vi "Add Topic.vi"(8 "error in (no error)":errorcluster, 9 "Topic Enqueuer":refnum<class "Message Enqueuer.lvclass">, 10 "Topic Object":refnum<class "Topic.lvclass">, 11 "TopicLookupTable":refnum<data-value>) -> (0 "error out":errorcluster, 2 "Topic Replaced?":bool, 3 "TopicLookupTable":refnum<data-value>)   [LabVIEW 2017, in "Mediator.lvlib" / "TopicLookupTable.lvclass"]
doc: "<License>\nCopyright © 2017 Composed Systems, LLC | All rights reserved\nwww.composed.io\n\nAuthor: Ethan Stern <ethan.stern@composed.io>\n\nThis software is provided \"AS IS\" WITHOUT WARRANTIES, either express or implied, AND IS FOR EDUCATIONAL PURPOSES ONLY.\n</License>"
uses:
  TopicLookupTable.lvclass
  Topic/Topic.lvclass
  <vilib>/ActorFramework/Message Enqueuer/Message Enqueuer.lvclass
  Topic/Topic.lvclass/Topic.ctl
  TopicLookupTable.lvclass/TopicLookupTable.ctl
  <vilib>/ActorFramework/Actor/Read Self Enqueuer.vi
  <vilib>/ActorFramework/Message Enqueuer/Init from Existing Queue.vi
  <vilib>/ErrorRing/Error Ring.xnode
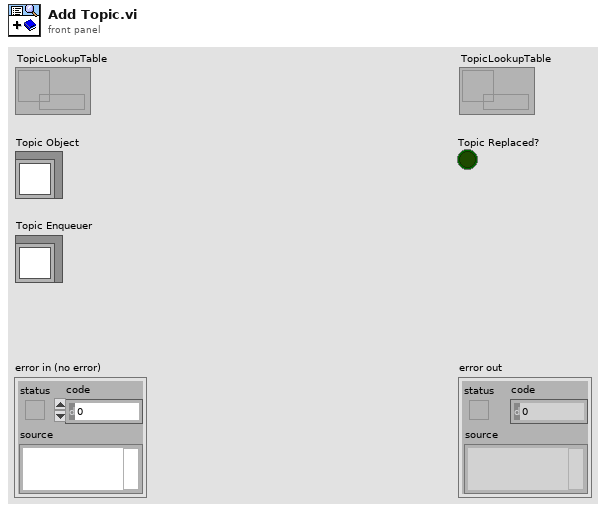
[diagram p1: front panel]
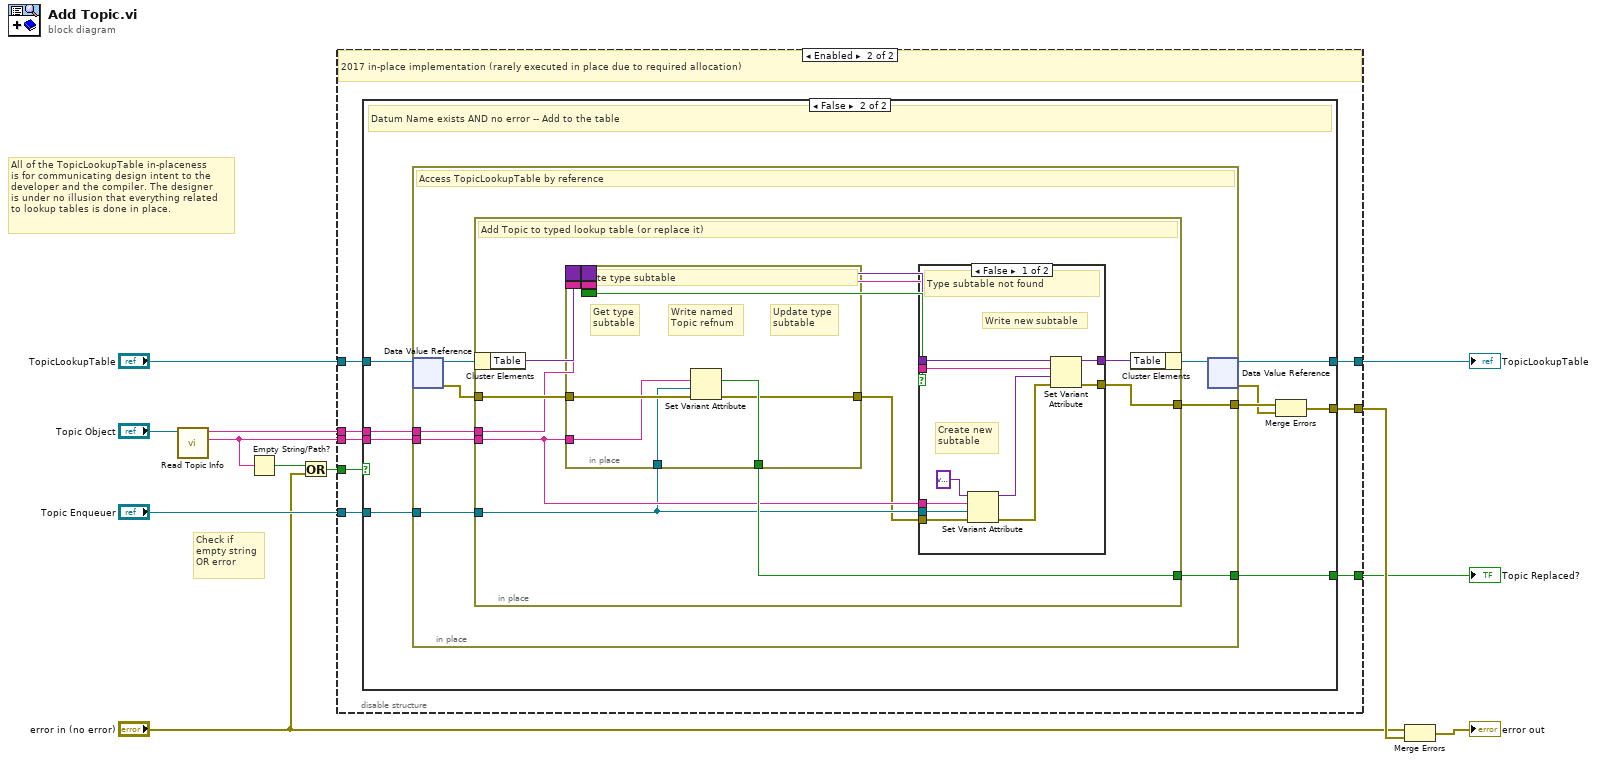
[diagram p0: block diagram]
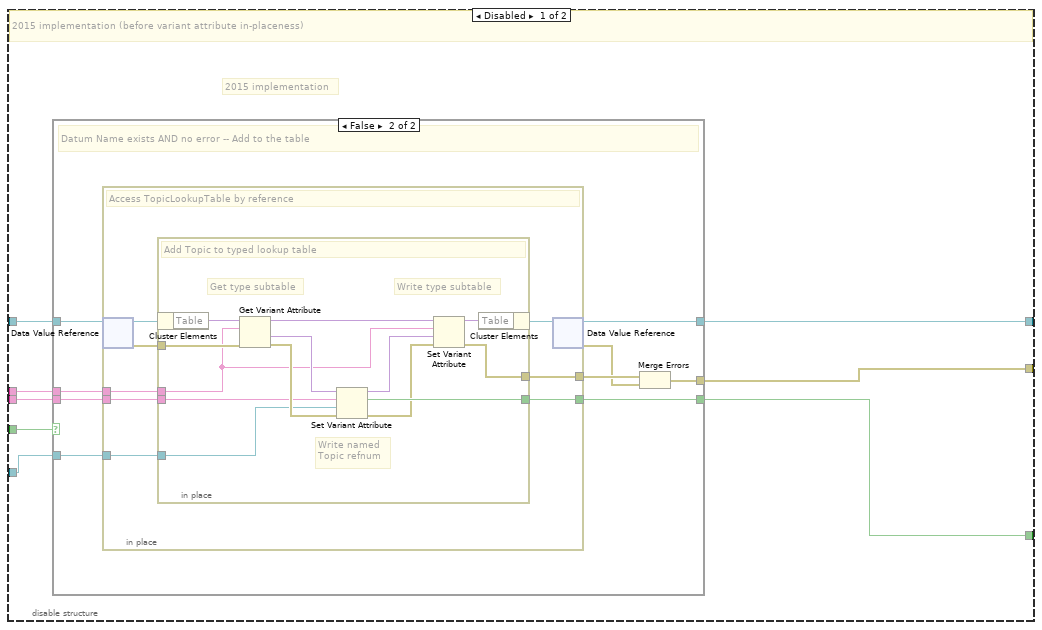
[diagram p2: hidden frame]
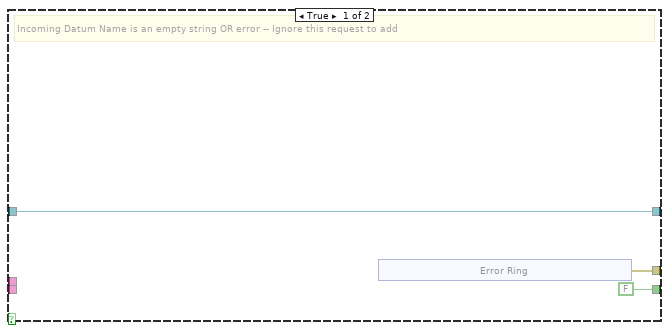
[diagram p3: hidden frame]
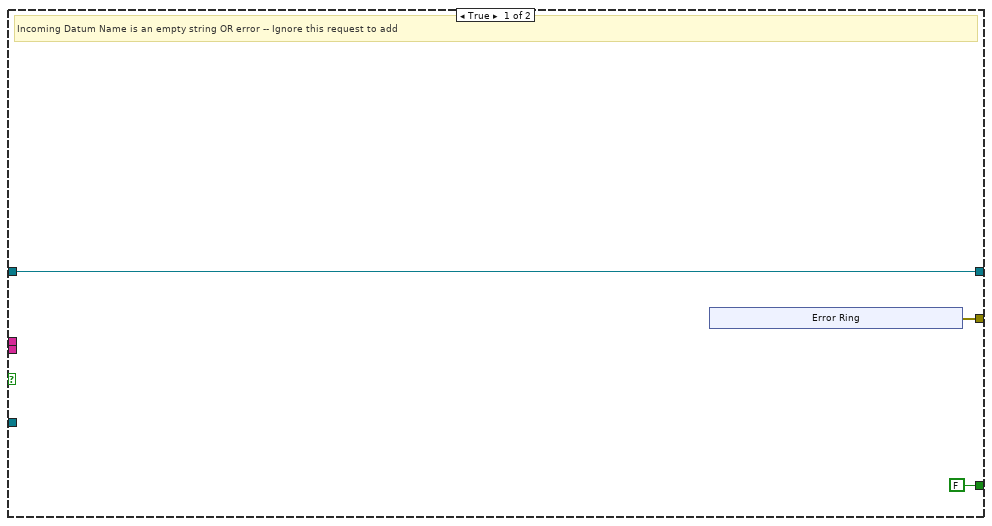
[diagram p4: hidden frame]
diagram:
  # "Check if\nempty string\nOR error"
  # "All of the TopicLookupTable in-placeness\nis for communicating design intent to the\ndeveloper and the compiler. The designer\nis under no illusion that everything related\nto lookup tables is done in place."
  n1 = call "Read Topic Info.vi"("Topic in"="Topic Object") -> ("Name"=w2:string, "Type"=w6:string)  [unwired: 7 in, 2 out]
  n2 = Empty String/Path?(string/path=w2) -> (empty?=w3:bool)
  n3 = Or(x=w3, y="error in (no error)") -> (x .or. y?=w1:bool)
  n4 = disable-structure shown="Enabled" {
    disable-tunnel: "TopicLookupTable" -> [w20 w62]
    disable-tunnel: [w19 w57] -> w10
    disable-tunnel: [w18 w55] -> w9
    disable-tunnel: "Topic Enqueuer" -> [w17 w58]
    disable-tunnel: w6 -> [w16 w59]
    disable-tunnel: [w15 w56] -> w5
    disable-tunnel: w2 -> [w14 w60]
    disable-tunnel: w1 -> [w13 w61]
    frame Disabled {
      # "2015 implementation"
      # "2015 implementation (before variant attribute in-placeness)"
      n5 = case shown="False" w13 {
        tunnel: w20 -> [w21 w29]
        tunnel: [w22 w28] -> w19
        tunnel: [FALSE ("replaced") w32] -> w18
        tunnel: w17 -> [_ w31]
        tunnel: w16 -> [_ w30]
        tunnel: [w21 w26] -> w15
        tunnel: w14 -> [_ w25]
        frame True {
          # "Incoming Datum Name is an empty string OR error -- Ignore this request to add"
          n6 = xnode "Error Ring"() -> ("error out"=w22:errorcluster)
        }
        frame False {
          # "Datum Name exists AND no error -- Add to the table"
          n7 = in-place {
            in-place-border: [w41] -> w33
            in-place-border: [w40] -> w32
            in-place-border: w31 -> [w39]
            in-place-border: w30 -> [w38]
            in-place-border: w25 -> [w37]
            # "Access TopicLookupTable by reference"
            n8 = in-place-dvr #1(w29) -> (w36:refnum<class "TopicLookupTable.lvclass">, w34:errorcluster)
            n9 = in-place {
              in-place-border: [w52] -> w41
              in-place-border: [w47] -> w40
              in-place-border: w39 -> [w45]
              in-place-border: w38 -> [w42]
              in-place-border: w37 -> [w44]
              in-place-border: w34 -> [w43]
              # "Write named\nTopic refnum"
              # "Write type subtable"
              # "Get type subtable"
              # "Add Topic to typed lookup table"
              n10 = in-place-cluster #2(w36) -> ("Table"=w51:variant)
              n11 = Get Variant Attribute(Variant=w51, name=w42, error in=w43) -> (duplicate Variant=w50:variant, value=w48:variant, error out=w54:errorcluster)  [unwired: 1 in, 1 out]
              n12 = Set Variant Attribute(Variant=w48, name=w44, value=w45, error in=w54) -> (Variant out=w49:variant, replaced=w47:bool, error out=w46:errorcluster)
              n13 = Set Variant Attribute(Variant=w50, name=w42, value=w49, error in=w46) -> (Variant out=w53:variant, error out=w52:errorcluster)  [unwired: 1 out]
              n14 = in-place-cluster #2("Table"=w53) -> (w35:refnum<class "TopicLookupTable.lvclass">)
            }
            n15 = in-place-dvr #1(w35) -> (w26:refnum<data-value>, w27:errorcluster)
          }
          n16 = Merge Errors(w33, w27) -> (w28:errorcluster)
        }
      }
    }
    frame Enabled {
      # "2017 in-place implementation (rarely executed in place due to required allocation)"
      n17 = case shown="False" w61 {
        tunnel: w62 -> [w63 w72]
        tunnel: [w64 w71] -> w57
        tunnel: [FALSE ("replaced") w75] -> w55
        tunnel: w58 -> [_ w74]
        tunnel: w59 -> [_ w73]
        tunnel: [w63 w70] -> w56
        tunnel: w60 -> [_ w69]
        frame True {
          # "Incoming Datum Name is an empty string OR error -- Ignore this request to add"
          n18 = xnode "Error Ring"() -> ("error out"=w64:errorcluster)
        }
        frame False {
          # "Datum Name exists AND no error -- Add to the table"
          n19 = in-place {
            in-place-border: [w83] -> w75
            in-place-border: w74 -> [w82]
            in-place-border: w73 -> [w81]
            in-place-border: w69 -> [w80]
            in-place-border: [w76] -> w68
            # "Access TopicLookupTable by reference"
            n20 = in-place-dvr #3(w72) -> (w79:refnum<class "TopicLookupTable.lvclass">, w77:errorcluster)
            n21 = in-place {
              in-place-border: [w94] -> w83
              in-place-border: w82 -> [w86]
              in-place-border: w81 -> [w92]
              in-place-border: w80 -> [w87]
              in-place-border: w77 -> [w95]
              in-place-border: [w84] -> w76
              # "Add Topic to typed lookup table (or replace it)"
              n22 = in-place-cluster #4(w79) -> ("Table"=w93:variant)
              n23 = in-place {
                in-place-border: [w100] -> w94
                in-place-border: w86 -> [w97]
                in-place-border: w87 -> [w98]
                border: w93 -> [_]
                border: w92 -> [_]
                border: [_] -> w90
                border: [_] -> w88
                border: [_] -> w91
                in-place-border: w95 -> [w102]
                in-place-border: [w96] -> w85
                # "Write named\nTopic refnum"
                # "Update type\nsubtable"
                # "Get type\nsubtable"
                # "Update type subtable"
                n24 = Set Variant Attribute(Variant=w99, name=w98, value=w97, error in=w102) -> (Variant out=w101:variant, replaced=w100:bool, error out=w96:errorcluster)
              }
              n25 = case shown="False" w91 {
                tunnel: w90 -> [w112 w114]
                tunnel: [w111 w114] -> w89
                tunnel: w88 -> [w110 _]
                tunnel: w87 -> [w109 _]
                tunnel: w86 -> [w108 _]
                tunnel: w85 -> [w104 w113]
                tunnel: [w103 w113] -> w84
                frame False {
                  # "Write new subtable"
                  # "Create new\nsubtable"
                  # "Type subtable not found"
                  n26 = Set Variant Attribute(Variant=variant ("variant"), name=w109, value=w108, error in=w104) -> (Variant out=w107:variant, error out=w105:errorcluster)  [unwired: 1 out]
                  n27 = Set Variant Attribute(Variant=w112, name=w110, value=w107, error in=w105) -> (Variant out=w111:variant, error out=w103:errorcluster)  [unwired: 1 out]
                }
                frame True {
                  # "Subtable updated okay"
                }
              }
              n28 = in-place-cluster #4("Table"=w89) -> (w78:refnum<class "TopicLookupTable.lvclass">)
            }
            n29 = in-place-dvr #3(w78) -> (w70:refnum<data-value>, w67:errorcluster)
          }
          n30 = Merge Errors(w68, w67) -> (w71:errorcluster)
        }
      }
    }
  }
  "Topic Replaced?" <- w9
  "TopicLookupTable" <- w5
  n31 = Merge Errors("error in (no error)", w10) -> (→"error out":errorcluster)
